vi "Set PointToRow.vi"(8 "error in (no error)":errorcluster caption="错误输入（无错误）", 10 "坐标":T1, 11 "listbox 输入":refnum<class "listbox.lvclass">) -> (0 "error out":errorcluster caption="错误输出", 2 "边界内？":bool, 3 "listbox 输出":refnum<class "listbox.lvclass">)   [LabVIEW 2016, in "listbox.lvclass"]
uses:
  listbox.lvclass
  <vilib>/Utility/miscctls.llb/LVPoint32TypeDef.ctl
  listbox.lvclass/listbox.ctl
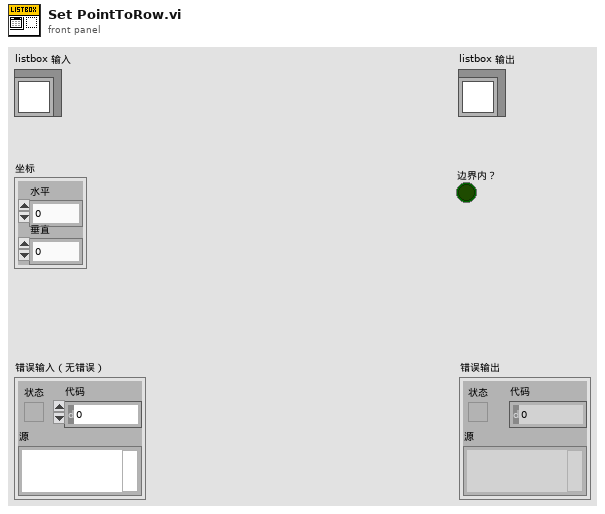
[diagram p1: front panel]
types:
  T1 = typedef "LVPoint32TypeDef.ctl" = cluster{"Horizontal":i32, "Vertical":i32}
  T2 = typedef "LVRowAndColumnTypeDef.ctl" = cluster{"Row":i32, "Column":i32}
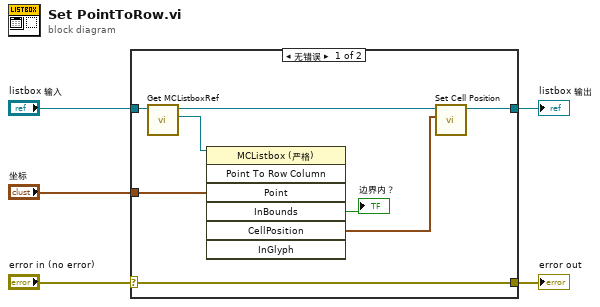
[diagram p0: block diagram]
diagram:
  n1 = case shown="无错误" "error in (no error)" {
    selector: "error in (no error)" -> [w12 w15]
    tunnel: [w12 w15] -> w4
    tunnel: [w8 w14] -> w2
    tunnel: "listbox 输入" -> [w13 w14]
    tunnel: "坐标" -> [w9 _]
    frame No Error {
      n2 = call "Get MCListboxRef.vi"("listbox in"=w13) -> ("MCListboxRef"=w10:refnum<vi>, "listbox out"=w11:refnum<class "listbox.lvclass">)  [unwired: 9 in]
      n3 = invoke class="MCListbox (严格)" method="Point To Row Column"(reference=w10, "Point"=w9) -> ("InBounds"=→"边界内？":bool, "CellPosition"=w6:T2)  [unwired: 5 in, 5 out]
      n4 = call "Set Cell Position.vi"("Cell Position"=w6, "listbox in"=w11) -> ("listbox out"=w8:refnum<class "listbox.lvclass">)  [unwired: 9 in]
    }
    frame Error {
    }
  }
  "error out" <- w4
  "listbox 输出" <- w2
